vi "SignalSenderLoop.SetSetpoint.vi"(8 "error in (no error)":errorcluster, 10 "Setpoint":dbl, 11 "SignalSenderLoop":refnum<class "SignalSenderLoop.lvclass">) -> (0 "error out":errorcluster, 3 "SignalSenderLoop out":refnum<class "SignalSenderLoop.lvclass">)   [LabVIEW 2020, in "ECU_Diagnose.lvlib" / "SignalSenderLoop.lvclass"]
doc: "---------------------------------------------------------------\nJKI State Machine Objects™\nhttp://jki.net/state-machine-objects/\nCopyright (C) 2005-2015, JKI <info@jki.net>\nALL RIGHTS RESERVEDJKI State Machine Objects (SMO) 1.0.0.5\nJKI - JKI\nCopyright (c) 2016, JKI"
uses:
  SignalSenderLoop.lvclass
  SignalSenderLoop.lvclass/SignalSenderLoop.ctl
  Typedefs/SetpointChanged--EventData--Cluster.ctl
  Typedefs/Data.ctl
panel:
  # "For instructions on how to use the JKI State Machine Objects, examples and video tutorials, visit:\nhttp://jki.net/state-machine-objects/\n\nJKI State Machine Objects™\nhttp://jki.net/state-machine-objects/\nCopyright (C) 2005-2015, JKI <info@jki.net>\nALL RIGHTS RESERVED"
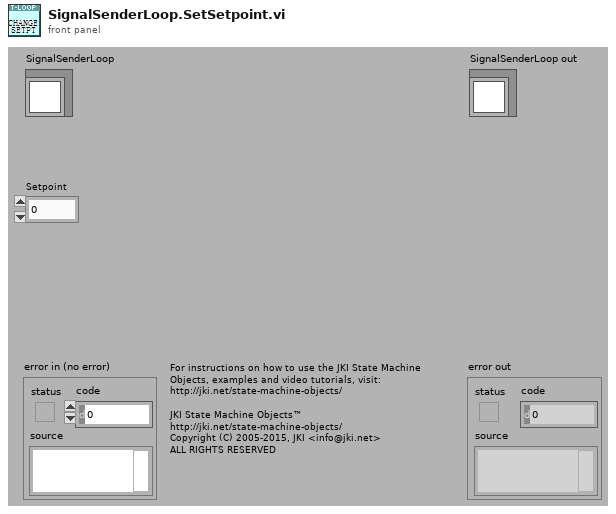
[diagram p1: front panel]
types:
  T1 = typedef "ECU_Diagnose.lvlib/SignalSenderLoop.lvclass/SetpointChanged--EventData--Cluster.ctl" = cluster{"Setpoint":T2}
  T2 = typedef "ECU_Diagnose.lvlib/SignalSenderLoop.lvclass/Data.ctl" = dbl
  T3 = typedef "ECU_Diagnose.lvlib/SignalSenderLoop.lvclass/PrivateData--Ref.ctl" = refnum<data-value>
  T4 = typedef "ECU_Diagnose.lvlib/SignalSenderLoop.lvclass/PrivateData--Cluster.ctl" = cluster{"Public Events":T5, "Setpoint":T2, "Private Events":T6, "SignalFrameSet":T7}
  T5 = typedef "ECU_Diagnose.lvlib/SignalSenderLoop.lvclass/PublicEvents--Cluster.ctl" = cluster{"Setpoint Changed":refnum<user-event>, "Value Changed":refnum<user-event>}
  T6 = typedef "ECU_Diagnose.lvlib/SignalSenderLoop.lvclass/PrivateEvents--Cluster.ctl" = cluster{"AsyncMethod":refnum<user-event>, "SignalCMDArry":refnum<user-event>}
  T7 = typedef "ECU_Diagnose.lvlib/SignalSenderLoop.lvclass/SignalFrameSet.ctl" = cluster{"Port_No.":refnum<k21>, "计数Count":bool, "校验CheckSum":bool, "MessageFrame":refnum<k21>, "校验算法名称":string}
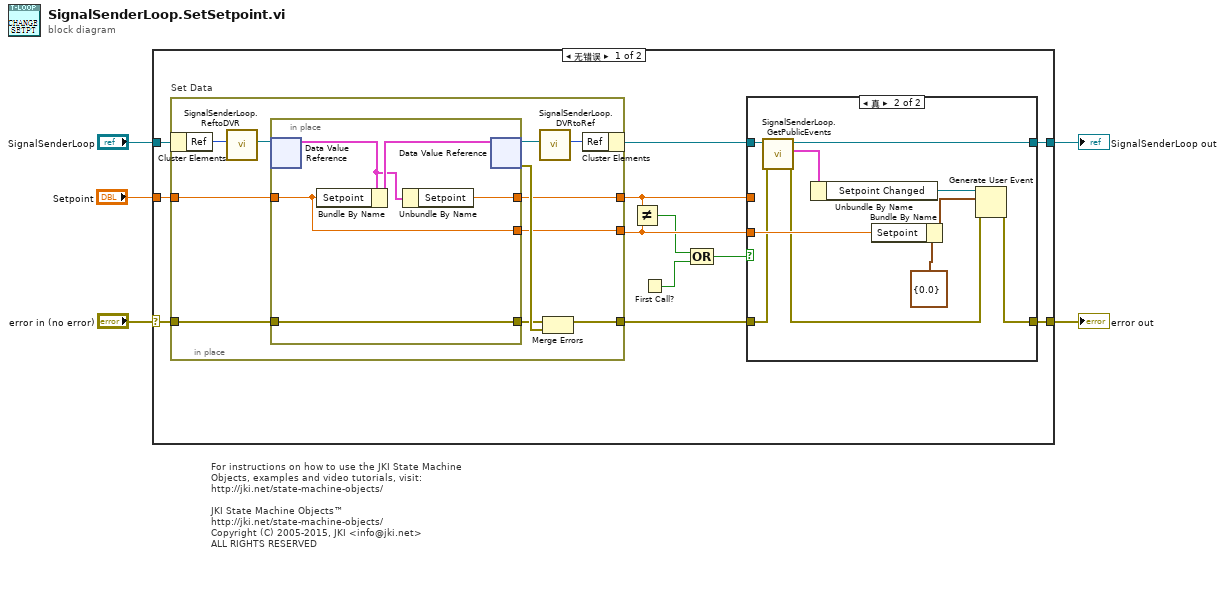
[diagram p0: block diagram]
diagram:
  # "For instructions on how to use the JKI State Machine Objects, examples and video tutorials, visit:\nhttp://jki.net/state-machine-objects/\n\nJKI State Machine Objects™\nhttp://jki.net/state-machine-objects/\nCopyright (C) 2005-2015, JKI <info@jki.net>\nALL RIGHTS RESERVED"
  n1 = case shown="无错误" "error in (no error)" {
    selector: "error in (no error)" -> [w15 w46]
    tunnel: "SignalSenderLoop" -> [w16 w47]
    tunnel: [w13 w46] -> w4
    tunnel: [w9 w47] -> w3
    tunnel: "Setpoint" -> [w17 _]
    frame No Error {
      n2 = in-place "Set Data" {
        in-place-border: w15 -> [w40]
        in-place-border: [w37] -> w14
        in-place-border: w17 -> [w36]
        in-place-border: [w35] -> w10
        in-place-border: [w34] -> w11
        n3 = in-place-cluster #1(w16) -> ("Ref"=w33:u32)
        n4 = call "SignalSenderLoop.ReftoDVR.vi"("Ref"=w33) -> ("Ref"=w32:T3)  [unwired: 10 in]
        n5 = in-place {
          in-place-border: w40 -> [w45]
          in-place-border: [w45] -> w38
          in-place-border: w36 -> [w43]
          in-place-border: [w43] -> w35
          in-place-border: [w42] -> w34
          n6 = in-place-dvr #2(w32) -> (w41:T4)  [unwired: 1 out]
          n7 = Bundle By Name(cluster=w41, "Setpoint"=w43) -> (w44:T4)
          n8 = Unbundle By Name(w41) -> ("Setpoint"=w42:T2)
          n9 = in-place-dvr #2(w44) -> (w31:T3, w39:errorcluster)
        }
        n10 = call "SignalSenderLoop.DVRtoRef.vi"("Ref"=w31) -> ("Ref"=w30:u32)  [unwired: 10 in]
        n11 = Merge Errors(w38, w39) -> (w37:errorcluster)
        n12 = in-place-cluster #1("Ref"=w30) -> (w12:refnum<class "SignalSenderLoop.lvclass">)
      }
      n13 = Not Equal?(x=w11, y=w10) -> (x != y?=w8:bool)
      n14 = First Call?() -> (First Call?: T/F=w7:bool)
      n15 = Compound Arithmetic op=OR(w8, w7) -> (w6:bool)
      n16 = case shown="真" w6 {
        tunnel: w14 -> [w18 w23]
        tunnel: w11 -> [_ _]
        tunnel: w10 -> [_ w26]
        tunnel: [w18 w25] -> w13
        tunnel: w12 -> [w19 w24]
        tunnel: [w19 w21] -> w9
        frame False {
        }
        frame True {
          n17 = call "SignalSenderLoop.GetPublicEvents.vi"("error in (no error)"=w23, "SignalSenderLoop"=w24) -> ("error out"=w22:errorcluster, "my Public Events"=w20:T5, "SignalSenderLoop out"=w21:refnum<class "SignalSenderLoop.lvclass">)  [unwired: 7 in]
          n18 = Unbundle By Name(w20) -> ("Setpoint Changed"=w29:refnum<user-event>)
          n19 = Bundle By Name(cluster=T1 {"Setpoint"=0.0} ("event data"), "Setpoint"=w26) -> (w27:T1)
          n20 = Generate User Event(user event=w29, event data cluster=w27, error in=w22) -> (error out=w25:errorcluster)  [unwired: 1 in, 1 out]
        }
      }
    }
    frame Error {
    }
  }
  "error out" <- w4
  "SignalSenderLoop out" <- w3
